vi "Compute_Number.vi"(8 "error in":errorcluster, 10 "Oscilloscope":cluster{"Record Len":i32, "Time Div":u16}={"Record Len"=4, "Time Div"=0} {"Time Div" items=["10m", "20ms", "50ms", "100ms", "200ms", "500ms", "1s", "2s", "5s", "10s", "20s", "30s", "1min", "2min", "5min"]; "Record Len" items=["10k", "25k", "50k", "100k", "250k", "500k", "1M", "2.5M", "5M", "10M", "25M", "50M", "100M", "250M", "500M", "1G", "2G", "4G", "5G", "10G", "20G", "50G"]}, 11 "Control Signal":T1={"Freq"=0.0, "level[V]"=0.0, "duty"=0.0, "On time[ms]"=50.0}) -> (0 "error out":errorcluster, 1 "output string":string, 2 "NumDiv":dbl, 3 "NumData":dbl)   [LabVIEW 2019]
uses:
  _ctrl/rw.ctl
  Durability/common/Global_params.vi
  Glob_Ref.vi
panel:
  in  "Time Division (12: 1ms)":i32(ring)=12 items=["100ns", "200ns", "500ns", "1us", "2us", "5us", "10us", "20us", "50us", "100us", "200us", "500us", "1ms", "2ms", "5ms", "10ms", "20ms", "50ms", "100ms", "200ms", "500ms", "1s", "2s", "3s", "4s", "5s", "6s", "10s", "20s", "30s", "1min", "2min", "3min", "4min", "5min", "6min", "10min", "12min", "30min", "1hour", "2hour", "3hour", "4hour", "5hour", "6hour", "8hour", "10hour", "12hour", "1day", "2day", "3day", "4day", "5day"]
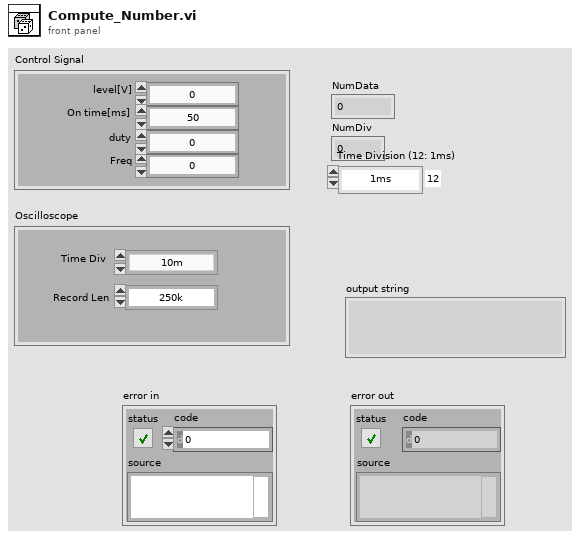
[diagram p1: front panel]
types:
  T1 = cluster{"Freq":dbl, "level[V]":dbl, "duty":dbl, "On time[ms]":dbl}
  T2 = typedef "rw.ctl" = enum16{"read", "write"}
  T3 = typedef "Testing-info.ctl" = cluster{"전체채널수":u8, "현재채널번호":u8, "Irms":dbl, "입력전압":dbl, "입력전류":dbl, "출력전압":dbl, "출력전류":dbl, "온도":dbl, "제어단 단선":bool, "제어단 단락":bool, "제어단 특성변화":bool, "출력단 단선":bool, "출력단 단락":bool, "출력단 특성변화":bool, "출력단 전압":bool, "카운트 일치":bool, "Irms 판정":bool, "온도":bool, "테스트 회수":u32, "TestType":T4, "현재회수":u32, "Ch selection":cluster{"1ch":bool, "2ch":bool, "3ch":bool, "4ch":bool, "5ch":bool, "6ch":bool}, "반복":u32, "Path":path, "파일생성주기":u32, "start time":dbl, "stop time":dbl, "현재반복회수":u32, "NG":cluster{"입출력 카운트":bool, "출력전류RMS":bool}}
  T4 = typedef "sequence_single.ctl" = enum16{"Register", "RC", "B1", "B2", "B3", "Oper_LV", "Oper_HV", "ContR_LV"}
  T5 = typedef "cDAQ-9269 Config.ctl" = cluster{"Ch":tag, "Max V":dbl, "Min V":dbl, " Rate":dbl, "N pts":i32, "sample mode":i32}
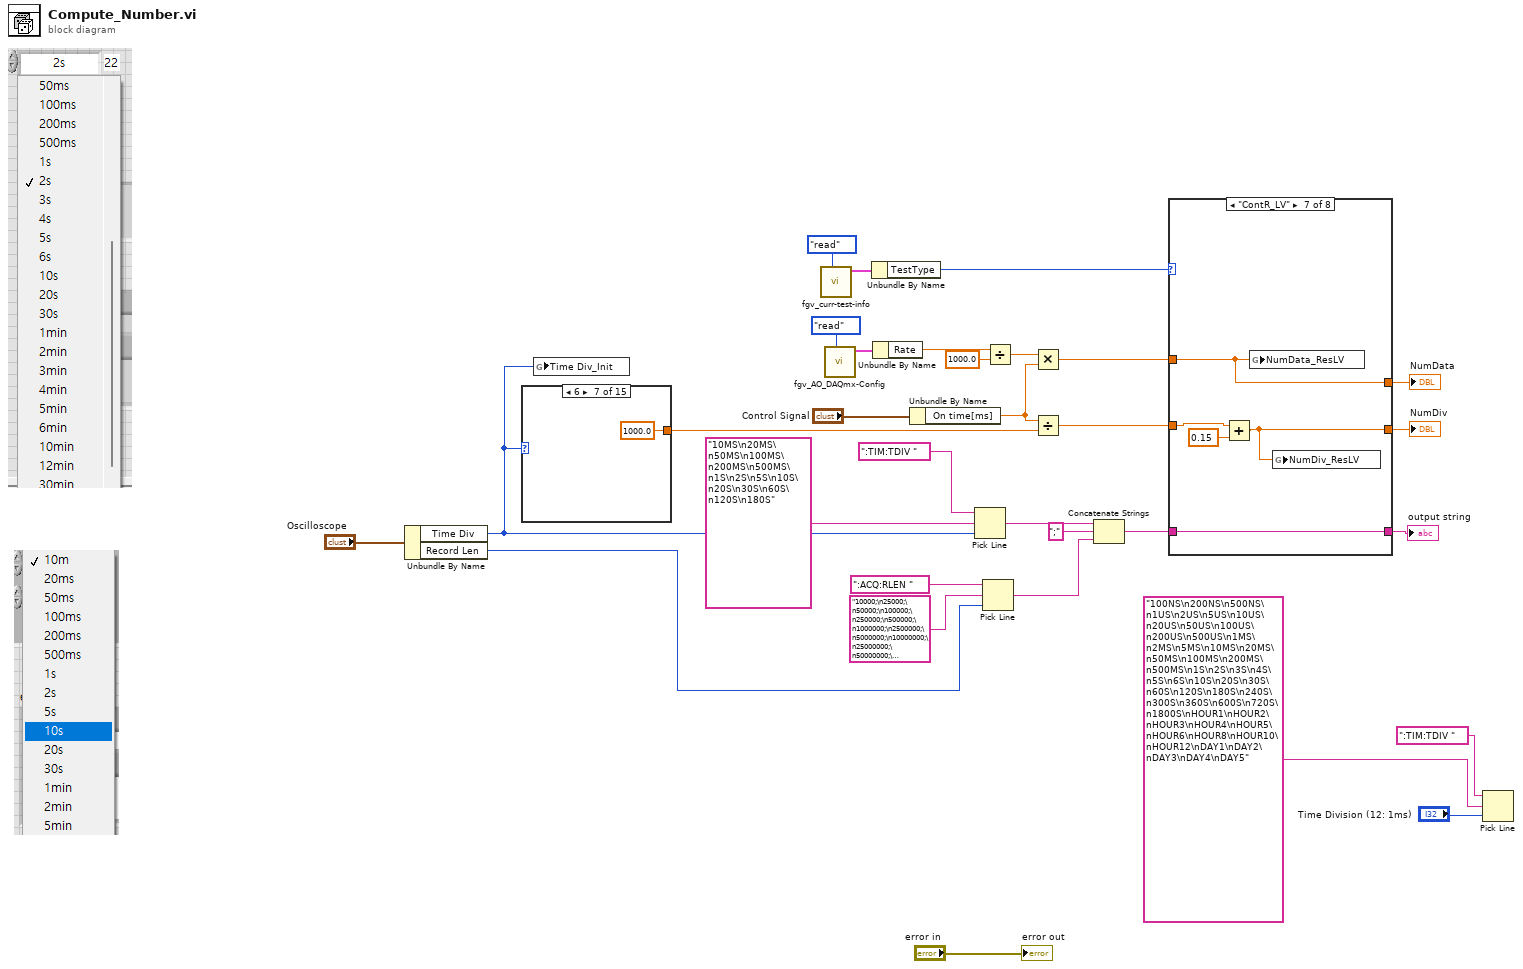
[diagram p0: block diagram]
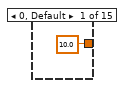
[diagram p2: hidden frame]
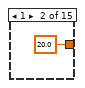
[diagram p3: hidden frame]
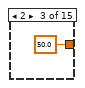
[diagram p4: hidden frame]
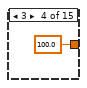
[diagram p5: hidden frame]
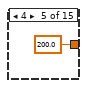
[diagram p6: hidden frame]
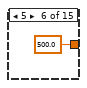
[diagram p7: hidden frame]
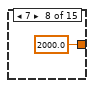
[diagram p8: hidden frame]
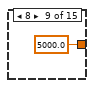
[diagram p9: hidden frame]
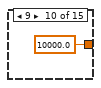
[diagram p10: hidden frame]
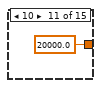
[diagram p11: hidden frame]
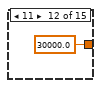
[diagram p12: hidden frame]
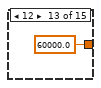
[diagram p13: hidden frame]
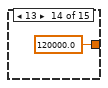
[diagram p14: hidden frame]
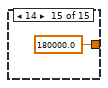
[diagram p15: hidden frame]
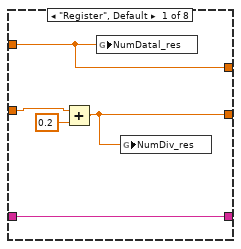
[diagram p16: hidden frame]
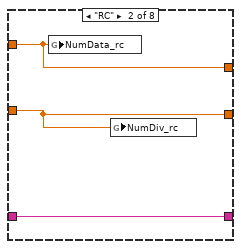
[diagram p17: hidden frame]
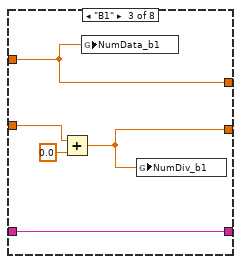
[diagram p18: hidden frame]
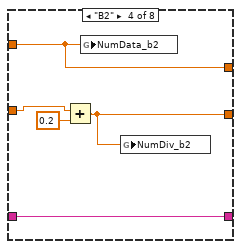
[diagram p19: hidden frame]
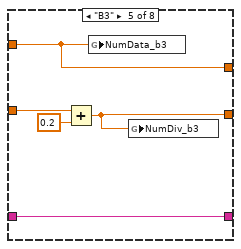
[diagram p20: hidden frame]
diagram:
  n1 = Unbundle By Name("Oscilloscope") -> ("Time Div"=w1:u16, "Record Len"=w27:i32)
  n2 = case shown="6" w1 {
    tunnel: [10.0 ("number") 20.0 ("number") 50.0 ("number") 100.0 ("number") 200.0 ("number") 500.0 ("number") 1000.0 ("number") 2000.0 ("number") 5000.0 ("number") 10000.0 ("number") 20000.0 ("number") 30000.0 ("number") 60000.0 ("number") 120000.0 ("number") 180000.0 ("number")] -> w2
    frame 0, Default {
    }
    frame 1 {
    }
    frame 2 {
    }
    frame 3 {
    }
    frame 4 {
    }
    frame 5 {
    }
    frame 6 {
    }
    frame 7 {
    }
    frame 8 {
    }
    frame 9 {
    }
    frame 10 {
    }
    frame 11 {
    }
    frame 12 {
    }
    frame 13 {
    }
    frame 14 {
    }
  }
  n3 = global write "Global_params.vi" "Time Div_Init"(w1) -> ()
  n4 = call "fgv_curr-test-info.vi"("cmd"=rw."read") -> ("현재테스트 정보 2"=w8:T3)  [unwired: 10 in]
  n5 = call "fgv_AO_DAQmx-Config.vi"("cmd"=rw."read") -> ("config 2"=w21:T5)  [unwired: 9 in, 1 out]
  n6 = Unbundle By Name(w8) -> ("TestType"=w7:T4)
  n7 = Unbundle By Name(w21) -> ("Rate"=w24:dbl)
  n8 = Unbundle By Name("Control Signal") -> ("On time[ms]"=w23:dbl)
  n9 = Pick Line ("ライン選択")(string ("")=":TIM:TDIV ", multi-line string="10MS\n20MS\n50MS\n100MS\n200MS\n500MS\n1S\n2S\n5S\n10S\n20S\n30S\n60S\n120S\n180S", line index=w1) -> (output string=w25:string)
  n10 = Pick Line ("ライン選択")(string ("")=":ACQ:RLEN ", multi-line string="10000;\n25000;\n50000;\n100000;\n250000;\n500000;\n1000000;\n2500000;\n5000000;\n10000000;\n25000000;\n50000000;\n100000000;\n250000000;\n500000000;\n1000000000;\n2000000000;\n4000000000;\n5000000000;\n10000000000;\n20000000000;\n50000000000;", line index=w27) -> (output string=w26:string)
  n11 = Divide(x=w24, y=1000.0) -> (x/y=w22:dbl)
  n12 = Multiply(x=w22, y=w23) -> (x*y=w13:dbl)
  n13 = Divide(x=w23, y=w2) -> (x/y=w6:dbl)
  n14 = Concatenate Strings(w25, ";" ("string"), w26) -> (w12:string)
  n15 = case shown="\"ContR_LV\"" w7 {
    tunnel: [w47 w52 w55 w60 w65 w70 w75 w80] -> w30
    tunnel: [w51 w54 w59 w64 w69 w74 w79 w82] -> w29
    tunnel: [w50 w53 w58 w63 w68 w73 w78 w81] -> w28
    tunnel: w13 -> [w51 w54 w59 w64 w69 w74 w79 w82]
    tunnel: w12 -> [w50 w53 w58 w63 w68 w73 w78 w81]
    tunnel: w6 -> [w48 w52 w56 w61 w66 w71 w76 w80]
    frame "Register", Default {
      n16 = Add(x=w48, y=0.2) -> (x+y=w47:dbl)
      n17 = global write "Glob_Ref.vi" "NumDatal_res"(w51) -> ()
      n18 = global write "Glob_Ref.vi" "NumDiv_res"(w47) -> ()
    }
    frame "RC" {
      n19 = global write "Glob_Ref.vi" "NumData_rc"(w54) -> ()
      n20 = global write "Glob_Ref.vi" "NumDiv_rc"(w52) -> ()
    }
    frame "B1" {
      n21 = Add(x=w56, y=0.0) -> (x+y=w55:dbl)
      n22 = global write "Glob_Ref.vi" "NumData_b1"(w59) -> ()
      n23 = global write "Glob_Ref.vi" "NumDiv_b1"(w55) -> ()
    }
    frame "B2" {
      n24 = Add(x=w61, y=0.2) -> (x+y=w60:dbl)
      n25 = global write "Glob_Ref.vi" "NumData_b2"(w64) -> ()
      n26 = global write "Glob_Ref.vi" "NumDiv_b2"(w60) -> ()
    }
    frame "B3" {
      n27 = Add(x=w66, y=0.2) -> (x+y=w65:dbl)
      n28 = global write "Glob_Ref.vi" "NumData_b3"(w69) -> ()
      n29 = global write "Glob_Ref.vi" "NumDiv_b3"(w65) -> ()
    }
    frame "Oper_LV" {
      n30 = Add(x=w71, y=0.15) -> (x+y=w70:dbl)
      n31 = global write "Glob_Ref.vi" "NumData_OLV"(w74) -> ()
      n32 = global write "Glob_Ref.vi" "NumDiv_OLV"(w70) -> ()
    }
    frame "ContR_LV" {
      n33 = Add(x=w76, y=0.15) -> (x+y=w75:dbl)
      n34 = global write "Glob_Ref.vi" "NumData_ResLV"(w79) -> ()
      n35 = global write "Glob_Ref.vi" "NumDiv_ResLV"(w75) -> ()
    }
    frame "Oper_HV" {
      n36 = global write "Glob_Ref.vi" "NumData_OHV"(w82) -> ()
      n37 = global write "Glob_Ref.vi" "NumDiv_OHV"(w80) -> ()
    }
  }
  "NumDiv" <- w30
  "NumData" <- w29
  "output string" <- w28
  n38 = Pick Line ("ライン選択")(string ("")=":TIM:TDIV ", multi-line string="100NS\n200NS\n500NS\n1US\n2US\n5US\n10US\n20US\n50US\n100US\n200US\n500US\n1MS\n2MS\n5MS\n10MS\n20MS\n50MS\n100MS\n200MS\n500MS\n1S\n2S\n3S\n4S\n5S\n6S\n10S\n20S\n30S\n60S\n120S\n180S\n240S\n300S\n360S\n600S\n720S\n1800S\nHOUR1\nHOUR2\nHOUR3\nHOUR4\nHOUR5\nHOUR6\nHOUR8\nHOUR10\nHOUR12\nDAY1\nDAY2\nDAY3\nDAY4\nDAY5", line index="Time Division (12: 1ms)") -> ()  [unwired: 1 out]
  "error out" <- "error in"
